vi "Examen (2).vi"() -> ()   [LabVIEW 2018]
panel:
  out "Array":bool[][](array[boolean])
  in  "stop":bool
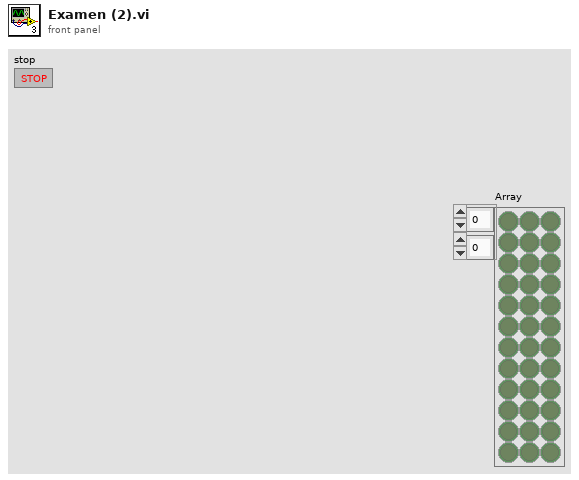
[diagram p1: front panel]
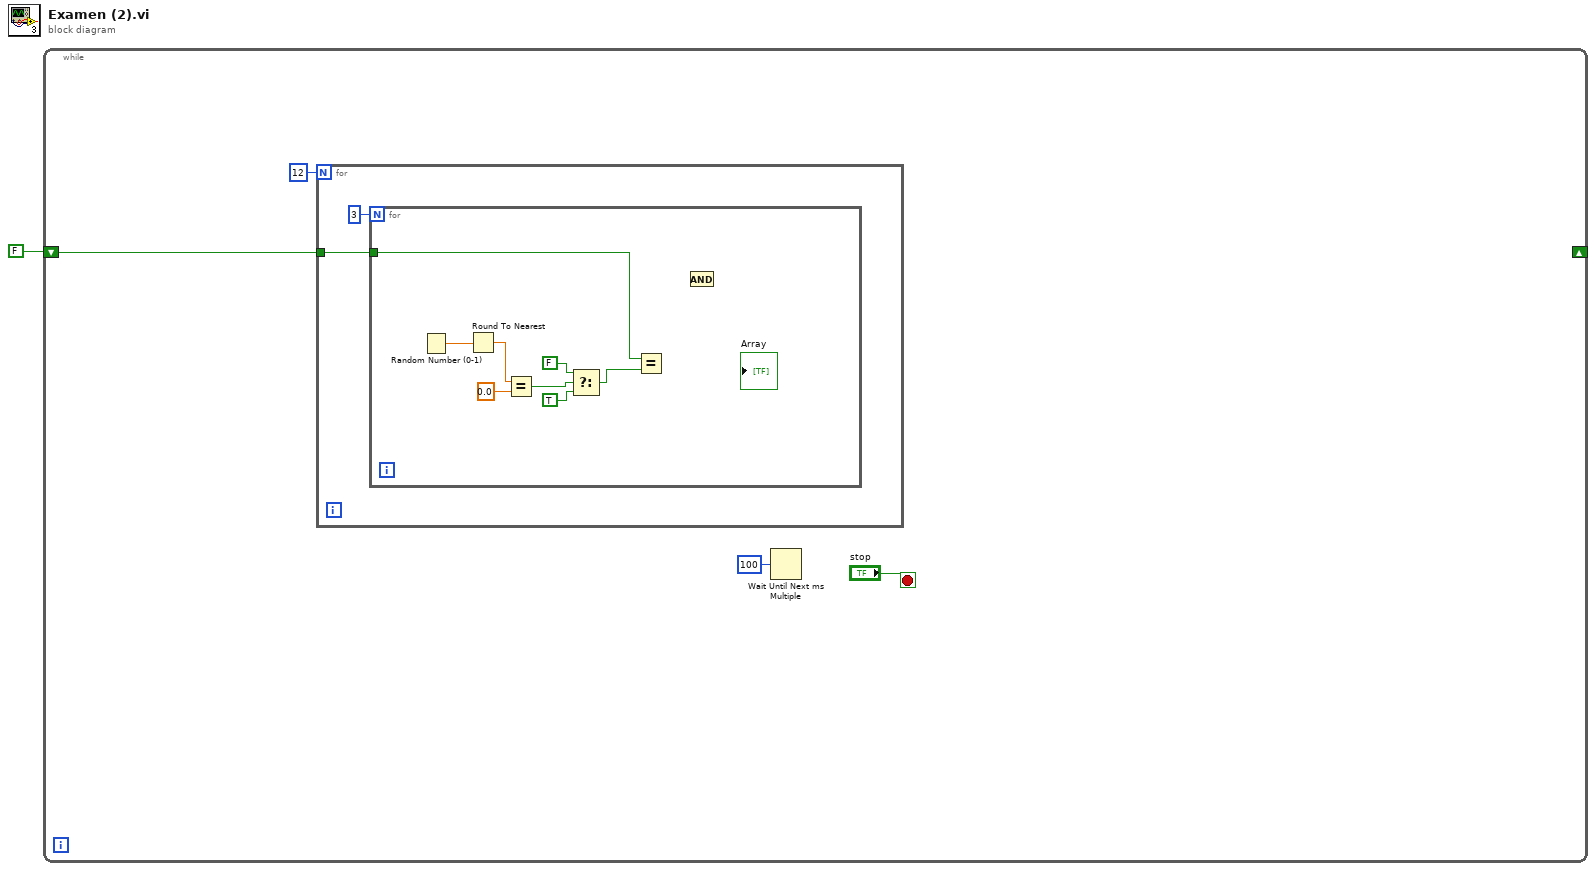
[diagram p0: block diagram]
diagram:
  n1 = while {
    shift-right: _ -> [_]
    shift-left: FALSE -> [w2]
    stop <- "stop" stop-if-true
    n2 = for {
      N: 12 -> [_]
      tunnel: w2 -> [w6]
      n3 = for {
        N: 3 -> [_]
        tunnel: w6 -> [w8]
        n4 = Random Number (0-1)() -> (number: 0 to 1=w15:dbl)
        n5 = Round To Nearest(number=w15) -> (nearest integer value=w14:dbl)
        n6 = Equal?(x=w14, y=0.0) -> (x = y?=w12:bool)
        n7 = Select(t=FALSE, s=w12, f=TRUE) -> (s? t:f=w9:bool)
        n8 = Equal?(x=w8, y=w9) -> ()  [unwired: 1 out]
        n9 = And() -> ()  [unwired: 2 in, 1 out]
      }
    }
    n10 = Wait Until Next ms Multiple(millisecond multiple=u32 100) -> ()  [unwired: 1 out]
  }
